vi "Voice Coil Voltage to FPGA Voltage.vi"(11 "Voltage In":dbl) -> (3 "Voltage Out":u16)   [LabVIEW 2018]
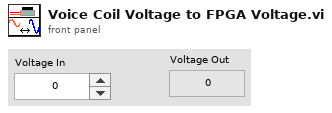
[diagram p1: front panel]
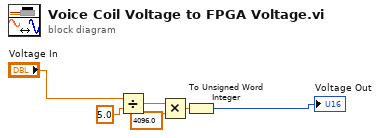
[diagram p0: block diagram]
diagram:
  n1 = Divide(x="Voltage In", y=5.0) -> (x/y=w5:dbl)
  n2 = Multiply(x=w5, y=4096.0) -> (x*y=w3:dbl)
  n3 = To Unsigned Word Integer(number=w3) -> (unsigned 16bit integer=→"Voltage Out":u16)
